vi "ex_5.vi"() -> ()   [LabVIEW 2020]
panel:
  out "Array/3 2":i32[](array[numeric])
  out "Array 2":i32[](array[numeric])
  in  "M 2":i32
  out "Array/3":i32[](array[numeric])
  out "Array":i32[](array[numeric])
  in  "M":i32
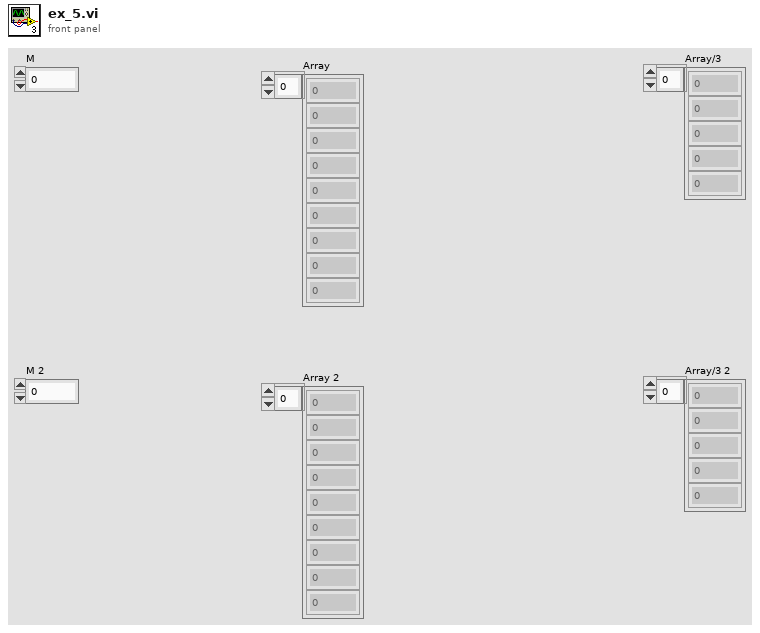
[diagram p1: front panel]
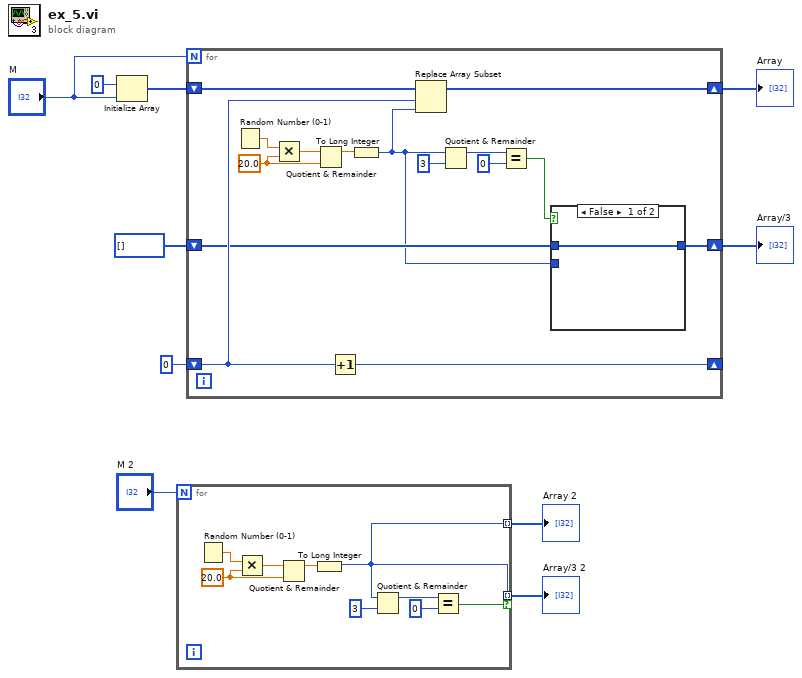
[diagram p0: block diagram]
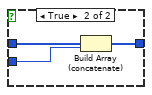
[diagram p2: hidden frame]
diagram:
  n1 = Initialize Array(0, "M") -> (w9:i32[])
  n2 = for {
    N: "M 2" -> [_]
    tunnel: [w12] -> w2 mode=indexing
    tunnel: [w12] -> w1 mode=indexing if=w11
    w17 = 20.0 ("y")
    n3 = Random Number (0-1)() -> (number: 0 to 1=w19:dbl)
    n4 = Multiply(x=w19, y=w17) -> (x*y=w18:dbl)
    n5 = Quotient & Remainder(x=w18, y=w17) -> (x-y*floor(x/y)=w16:dbl)  [unwired: 1 out]
    n6 = To Long Integer(number=w16) -> (32bit integer=w12:i32)
    n7 = Quotient & Remainder(x=w12, y=3) -> (x-y*floor(x/y)=w14:i32)  [unwired: 1 out]
    n8 = Equal?(x=w14, y=0) -> (x = y?=w11:bool)
  }
  "Array 2" <- w2
  "Array/3 2" <- w1
  n9 = for {
    N: "M" -> [_]
    shift-right: [w27] -> w7
    shift-left: w9 -> [w34]
    shift-right: [w33] -> _
    shift-left: 0 -> [w28]
    shift-right: [w20] -> w4
    shift-left: i32[] [] -> [w25]
    w30 = 20.0 ("y")
    n10 = Random Number (0-1)() -> (number: 0 to 1=w32:dbl)
    n11 = Multiply(x=w32, y=w30) -> (x*y=w31:dbl)
    n12 = Quotient & Remainder(x=w31, y=w30) -> (x-y*floor(x/y)=w29:dbl)  [unwired: 1 out]
    n13 = Increment(x=w28) -> (x+1=w33:i32)
    n14 = To Long Integer(number=w29) -> (32bit integer=w21:i32)
    n15 = Replace Array Subset(array=w34, new element=w21, index=w28) -> (w27:i32[])
    n16 = Quotient & Remainder(x=w21, y=3) -> (x-y*floor(x/y)=w24:i32)  [unwired: 1 out]
    n17 = Equal?(x=w24, y=0) -> (x = y?=w22:bool)
    n18 = case shown="False" w22 {
      tunnel: w25 -> [w35 w38]
      tunnel: w21 -> [_ w37]
      tunnel: [w35 w36] -> w20
      frame False {
      }
      frame True {
        n19 = Build Array (concatenate)(w38, w37) -> (w36:i32[])
      }
    }
  }
  "Array" <- w7
  "Array/3" <- w4
